vi "UART Write.vi"() -> ()   [LabVIEW 2020, in "CTI-Scratchpad.lvlib"]
uses:
  CTI-Scratchpad.lvlib
  CTI/UART Number.ctl
  CTI/GPIO Number.ctl
  CTI/Session/Session.lvclass
  CTI/VisaComms/VisaComms.lvclass
  CTI/CTI.lvlib
panel:
  in  "RX GPIO":T1=1
  in  "TX GPIO":T1
  in  "Baud":u32=19200
  in  "UART":T2
  in  "Write":bool
  in  "Data":string="Hello, world!"
  in  "stop":bool
  in  "Port":refnum<visa-resource-name>="COM3"
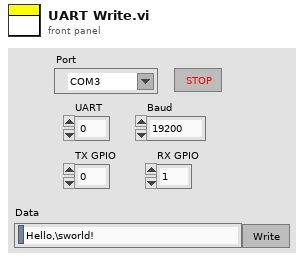
[diagram p1: front panel]
types:
  T1 = typedef "CTI.lvlib/GPIO Number.ctl" = i8
  T2 = typedef "CTI.lvlib/UART Number.ctl" = i8
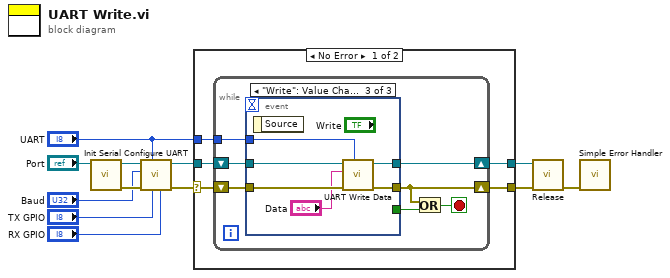
[diagram p0: block diagram]
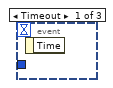
[diagram p2: hidden frame]
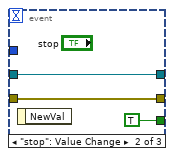
[diagram p3: hidden frame]
diagram:
  n1 = call "Init Serial.vi"("VISA resource name in"="Port") -> ("error out"=w10:errorcluster, "Session"=w11:refnum<class "Session.lvclass">)  [unwired: 8 in, 1 out]
  n2 = call "Configure UART.vi"("RX GPIO"="RX GPIO", "TX GPIO"="TX GPIO", "UART #"="UART", "error in (no error)"=w10, "Baud"="Baud", "Session in"=w11) -> ("error out"=w9:errorcluster, "Session out"=w8:refnum<class "Session.lvclass">)  [unwired: 4 in]
  n3 = case shown="No Error" w9 {
    selector: w9 -> [w15 w35]
    tunnel: w8 -> [w16 w34]
    tunnel: "UART" -> [w17 _]
    tunnel: [w14 w35] -> w7
    tunnel: [w13 w34] -> w6
    frame No Error {
      n4 = while {
        tunnel: w17 -> [w23]
        shift-right: [w22] -> w13
        shift-left: w16 -> [w24]
        shift-right: [w20] -> w14
        shift-left: w15 -> [w21]
        stop <- w18 stop-if-true
        n5 = event shown="[2] \"Write\": Value Change" {
          selector: _ -> [_ _ _]
          dyn-events: _ -> [_ _ _]
          timeout: _ -> [_ _ _]
          tunnel: w24 -> [_ w27 w33]
          tunnel: w23 -> [_ _ w29]
          tunnel: [_ w27 w31] -> w22
          tunnel: w21 -> [_ w26 w32]
          tunnel: [_ w26 w30] -> w20
          tunnel: [_ TRUE _] -> w19
          event Timeout {
            n6 = event-data() -> ()  [unwired: 1 in, 1 out]
          }
          event "stop": Value Change {
            n7 = event-data() -> ()  [unwired: 1 in, 1 out]
          }
          event "Write": Value Change {
            n8 = event-data() -> ()  [unwired: 1 in, 1 out]
            n9 = call "UART Write Data.vi"("UART #"=w29, "error in (no error)"=w32, "Data"="Data", "Session in"=w33) -> ("error out"=w30:errorcluster, "Session out"=w31:refnum<class "Session.lvclass">)  [unwired: 6 in]
          }
        }
        n10 = Or(x=w20, y=w19) -> (x .or. y?=w18:bool)
      }
    }
    frame Error {
    }
  }
  n11 = call-dynamic "Release.vi"("error in (no error)"=w7, "Session in"=w6) -> ("error out"=w5:errorcluster)  [unwired: 9 in]
  n12 = call <vilib>:"Simple Error Handler.vi"("error in (no error)"=w5) -> ()  [unwired: 4 in, 5 out]
